vi "Clear UI.vi"(11 "Table":refnum<vi>) -> ()   [LabVIEW 2017]
uses:
  <vilib>/Utility/miscctls.llb/LVRowAndColumnTypeDef.ctl
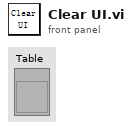
[diagram p1: front panel]
types:
  T1 = typedef "LVRowAndColumnTypeDef.ctl" = cluster{"Row":i32, "Column":i32}
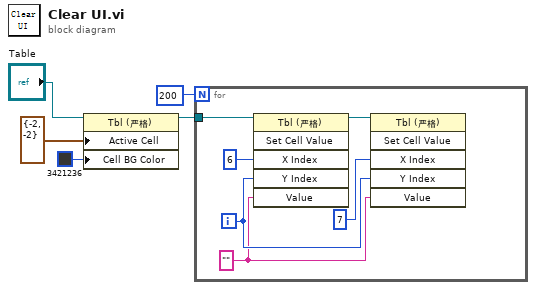
[diagram p0: block diagram]
diagram:
  n1 = property class="Tbl (严格)"(reference="Table", "Active Cell"=T1 {"Row"=-2, "Column"=-2} ("活动单元格:活动单元格"), "Cell BG Color"=u32 3421236) -> (reference out=w3:refnum<vi>)  [unwired: 1 in, 1 out]
  n2 = for {
    N: 200 -> [_]
    tunnel: w3 -> [w8]
    i -> [w7]
    w6 = ""
    n3 = invoke class="Tbl (严格)" method="Set Cell Value"(reference=w8, "X Index"=6 ("Y索引"), "Y Index"=w7, "Value"=w6) -> (reference out=w11:refnum<vi>)  [unwired: 2 in, 5 out]
    n4 = invoke class="Tbl (严格)" method="Set Cell Value"(reference=w11, "X Index"=7 ("Y索引"), "Y Index"=w7, "Value"=w6) -> ()  [unwired: 2 in, 6 out]
  }
